vi "Set pin status.vi"(7 "Value":bool, 8 "error in (no error)":errorcluster, 9 "Pin":dbl, 10 "Port":dbl, 11 "Arduino in":refnum<class "Arduino.lvclass">) -> (0 "error out":errorcluster, 3 "Arduino out":refnum<class "Arduino.lvclass">)   [LabVIEW 2020, in "Arduino.lvclass"]
doc: "Override del papa Set pin Status"
uses:
  Arduino.lvclass
  291d468d-7481-47cf-b55e-ac65055b3669.vi
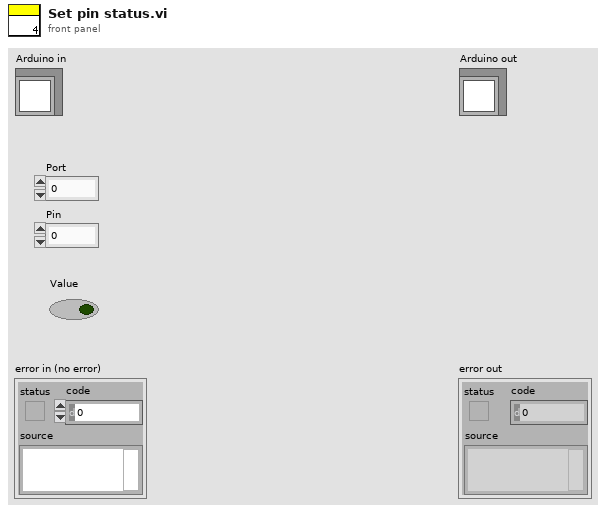
[diagram p1: front panel]
types:
  T1 = typedef "Serial Device.lvclass/serial device brand.ctl" = string
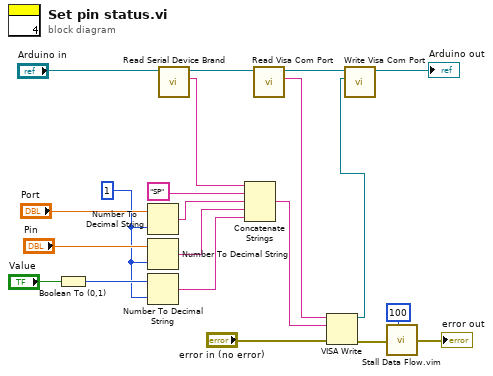
[diagram p0: block diagram]
diagram:
  w15 = i16 1 ("width (-)")
  n1 = Boolean To (0,1)(Boolean="Value") -> (0, 1=w16:i16)
  n2 = Number To Decimal String(number="Port", width (-)=w15) -> (decimal integer string=w12:string)
  n3 = Number To Decimal String(number="Pin", width (-)=w15) -> (decimal integer string=w11:string)
  n4 = Number To Decimal String(number=w16, width (-)=w15) -> (decimal integer string=w10:string)
  n5 = call-dynamic "Read Serial Device Brand.vi"("Serial Device in"="Arduino in") -> ("Serial Device Brand"=w14:T1, "Serial Device out"=w20:refnum<class "Arduino.lvclass">)  [unwired: 8 in, 1 out]
  n6 = Concatenate Strings(w14, "SP" ("string"), w12, w11, w10) -> (w9:string)
  n7 = call-dynamic "Read Visa Com Port.vi"("Serial Device in"=w20) -> ("Visa Com Port"=w8:string, "Serial Device out"=w7:refnum<class "Arduino.lvclass">)  [unwired: 8 in, 1 out]
  n8 = VISA Write(VISA resource name=w8, write buffer=w9, error in (no error)="error in (no error)") -> (VISA resource name out=w1:refnum<visa-resource-name>, error out=w4:errorcluster)  [unwired: 1 out]
  n9 = call-dynamic "Write Visa Com Port.vi"("Visa Com Port"=w1, "Serial Device in"=w7) -> ("Serial Device out"=→"Arduino out":refnum<class "Arduino.lvclass">)  [unwired: 8 in, 1 out]
  n10 = call "Stall Data Flow.vim"("value in"=w4, "milliseconds to wait"=u32 100) -> ("value out"=→"error out":errorcluster)  [unwired: 1 out]
